vi "Check slice image.vi"(8 "Error in":errorcluster, 9 "Pause?":bool[](array[boolean]), 10 "image thickness":u32[](array[numeric]), 11 "slice thickness":u32[](array[numeric])) -> (0 "Error out":errorcluster, 5 "Exit?":bool)   [LabVIEW 2018]
uses:
  Controls/Queue Manager Actions.ctl
  Controls/MessagePacket.ctl
  Controls/FGV Actions.ctl
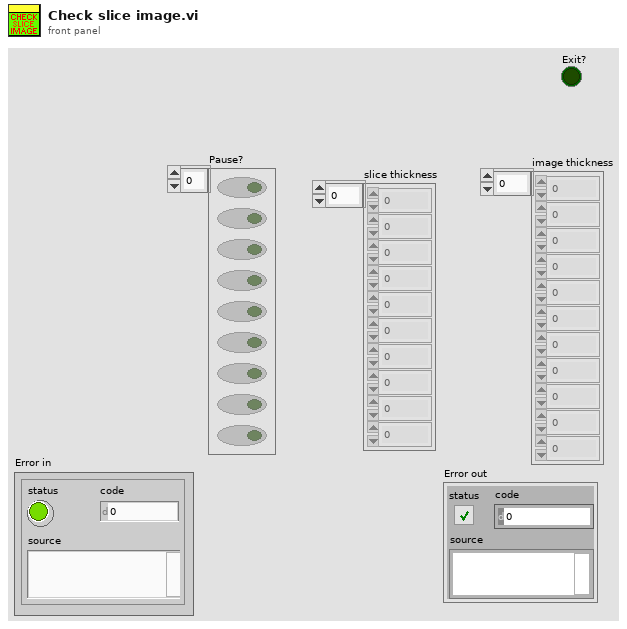
[diagram p1: front panel]
types:
  T1 = typedef "FGV Actions.ctl" = enum16{"Init", "Set", "Get", "Clear"}
  T2 = typedef "Queue Manager Actions.ctl" = enum16{"Init", "Enqueue", "Enqueue All", "Preview Queue", "Dequeue", "Get Status", "Flush Queue", "Flush All Queues", "Release All Queues", "Release Queue", "Enqueue at Opposite End"}
  T3 = typedef "MessagePacket.ctl" = cluster{"Message":string, "Parameter":variant}
  T4 = typedef "ScanType.ctl" = enum16{"Single Frame", "Continuous Frame", "ROI Line", "Vibratome", "Mosaic", "Mosaic + Slice"}
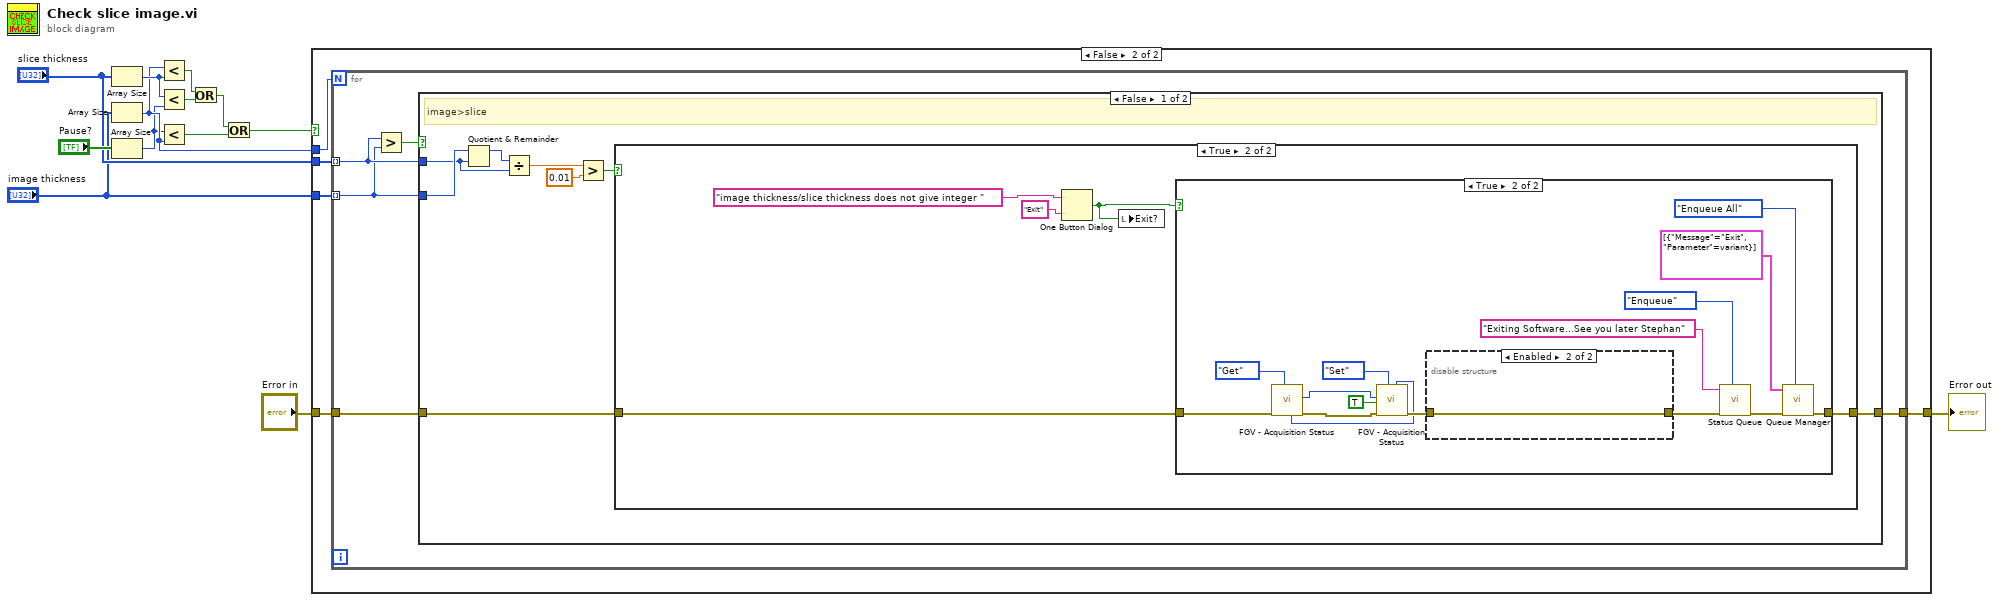
[diagram p0: block diagram]
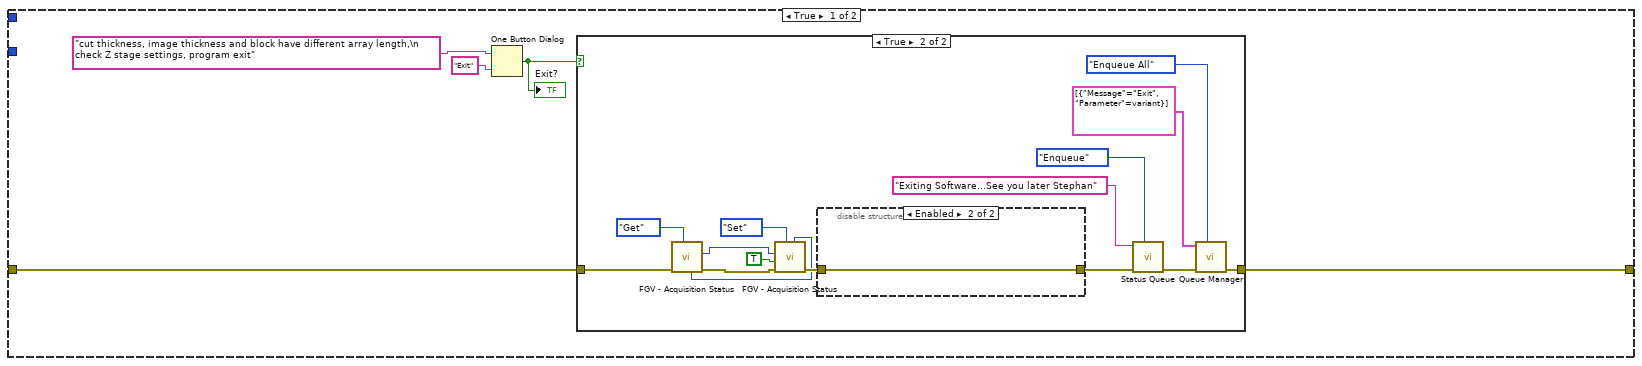
[diagram p2: hidden frame]
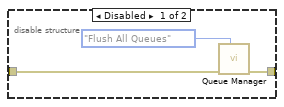
[diagram p4: hidden frame]
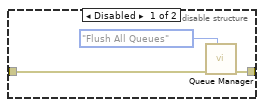
[diagram p7: hidden frame]
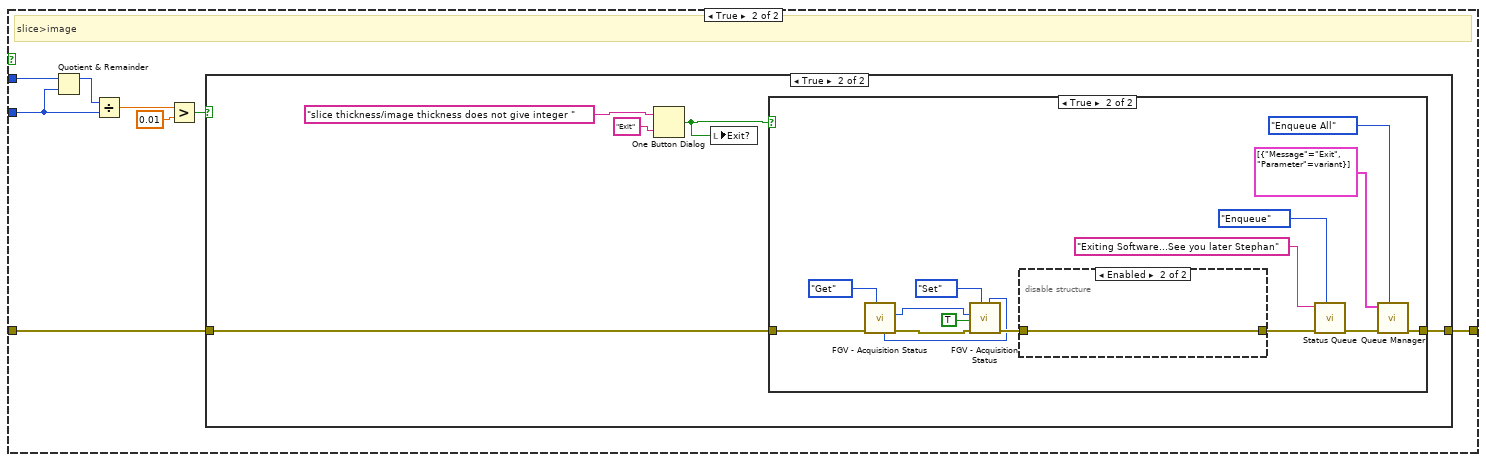
[diagram p8: hidden frame]
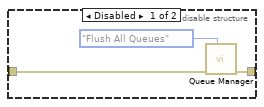
[diagram p11: hidden frame]
diagram:
  n1 = Array Size(array="slice thickness") -> (size(s)=w5:i32)
  n2 = Array Size(array="image thickness") -> (size(s)=w4:i32)
  n3 = Array Size(array="Pause?") -> (size(s)=w3:i32)
  n4 = Less?(x=w4, y=w5) -> (x < y?=w11:bool)
  n5 = Less?(x=w5, y=w3) -> (x < y?=w10:bool)
  n6 = Less?(x=w3, y=w4) -> (x < y?=w7:bool)
  n7 = Or(x=w11, y=w10) -> (x .or. y?=w8:bool)
  n8 = Or(x=w8, y=w7) -> (x .or. y?=w6:bool)
  n9 = case shown="False" w6 {
    tunnel: "Error in" -> [w15 w40]
    tunnel: [w14 w39] -> w12
    tunnel: w4 -> [_ w43]
    tunnel: "slice thickness" -> [_ w42]
    tunnel: "image thickness" -> [_ w41]
    frame True {
      n10 = One Button Dialog(message="cut thickness, image thickness and block have different array length,\n check Z stage settings, program exit", button name ("OK")="Exit") -> (true=w16:bool)
      "Exit?" <- w16
      n11 = case shown="True" w16 {
        tunnel: w15 -> [w19 w21]
        tunnel: [w19 w20] -> w14
        frame False {
        }
        frame True {
          n12 = call "FGV - Acquisition Status.vi"("Actions"=FGV_Actions."Get", "Error In"=w21) -> ("Error Out"=w26:errorcluster, "Scan Type [Out]"=w24:T4, "mem loc out"=w22:i32)  [unwired: 6 in, 1 out]
          n13 = call "FGV - Acquisition Status.vi"("mem loc"=w22, "Actions"=FGV_Actions."Set", "Error In"=w26, "Quit status"=TRUE, "Scan Type [In]"=w24) -> ("Error Out"=w25:errorcluster)  [unwired: 3 in, 3 out]
          n14 = disable-structure shown="Enabled" {
            disable-tunnel: [w36 w38] -> w29
            disable-tunnel: w25 -> [w35 w38]
            frame Disabled {
              n15 = call "Queue Manager.vi"("Action"=Queue_Manager_Actions."Flush All Queues", "Error In"=w35) -> ("Error Out"=w36:errorcluster)  [unwired: 5 in, 4 out]
            }
            frame Enabled {
            }
          }
          n16 = call "Status Queue.vi"("Action"=Queue_Manager_Actions."Enqueue", "Error In"=w29, "Status Message [In]"="Exiting Software...See you later Stephan") -> ("Error Out"=w31:errorcluster)  [unwired: 7 in, 1 out]
          n17 = call "Queue Manager.vi"("Action"=Queue_Manager_Actions."Enqueue All", "Error In"=w31, "Message Packet Array"=T3[] [{"Message"="Exit", "Parameter"=variant}] ("Message Packet [In]")) -> ("Error Out"=w20:errorcluster)  [unwired: 4 in, 4 out]
        }
      }
    }
    frame False {
      n18 = for {
        N: w43 -> [_]
        tunnel: w42 -> [w47] mode=indexing
        tunnel: w41 -> [w46] mode=indexing
        tunnel: w40 -> [w45]
        tunnel: [w44] -> w39
        n19 = Greater?(x=w47, y=w46) -> (0:w48:bool)
        n20 = case shown="False" w48 {
          tunnel: w47 -> [w50 w90]
          tunnel: w46 -> [w51 w85]
          tunnel: w45 -> [w52 w87]
          tunnel: [w49 w83] -> w44
          frame False {
            # "image>slice"
            n21 = Quotient & Remainder(x=w51, y=w50) -> (x-y*floor(x/y)=w54:u32)  [unwired: 1 out]
            n22 = Divide(x=w54, y=w50) -> (x/y=w53:dbl)
            n23 = Greater?(x=w53, y=0.01) -> (0:w55:bool)
            n24 = case shown="True" w55 {
              tunnel: w52 -> [w57 w60]
              tunnel: [w57 w59] -> w49
              frame False {
              }
              frame True {
                n25 = One Button Dialog(message="image thickness/slice thickness does not give integer ", button name ("OK")="Exit") -> (true=w58:bool)
                n26 = local write "Exit?"(w58) -> ()
                n27 = case shown="True" w58 {
                  tunnel: w60 -> [w63 w65]
                  tunnel: [w63 w64] -> w59
                  frame False {
                  }
                  frame True {
                    n28 = call "FGV - Acquisition Status.vi"("Actions"=FGV_Actions."Get", "Error In"=w65) -> ("Error Out"=w70:errorcluster, "Scan Type [Out]"=w68:T4, "mem loc out"=w66:i32)  [unwired: 6 in, 1 out]
                    n29 = call "FGV - Acquisition Status.vi"("mem loc"=w66, "Actions"=FGV_Actions."Set", "Error In"=w70, "Quit status"=TRUE, "Scan Type [In]"=w68) -> ("Error Out"=w69:errorcluster)  [unwired: 3 in, 3 out]
                    n30 = disable-structure shown="Enabled" {
                      disable-tunnel: [w80 w82] -> w73
                      disable-tunnel: w69 -> [w79 w82]
                      frame Disabled {
                        n31 = call "Queue Manager.vi"("Action"=Queue_Manager_Actions."Flush All Queues", "Error In"=w79) -> ("Error Out"=w80:errorcluster)  [unwired: 5 in, 4 out]
                      }
                      frame Enabled {
                      }
                    }
                    n32 = call "Status Queue.vi"("Action"=Queue_Manager_Actions."Enqueue", "Error In"=w73, "Status Message [In]"="Exiting Software...See you later Stephan") -> ("Error Out"=w75:errorcluster)  [unwired: 7 in, 1 out]
                    n33 = call "Queue Manager.vi"("Action"=Queue_Manager_Actions."Enqueue All", "Error In"=w75, "Message Packet Array"=T3[] [{"Message"="Exit", "Parameter"=variant}] ("Message Packet [In]")) -> ("Error Out"=w64:errorcluster)  [unwired: 4 in, 4 out]
                  }
                }
              }
            }
          }
          frame True {
            # "slice>image"
            n34 = Quotient & Remainder(x=w90, y=w85) -> (x-y*floor(x/y)=w86:u32)  [unwired: 1 out]
            n35 = Divide(x=w86, y=w85) -> (x/y=w84:dbl)
            n36 = Greater?(x=w84, y=0.01) -> (0:w88:bool)
            n37 = case shown="True" w88 {
              tunnel: w87 -> [w91 w93]
              tunnel: [w91 w92] -> w83
              frame False {
              }
              frame True {
                n38 = One Button Dialog(message="slice thickness/image thickness does not give integer ", button name ("OK")="Exit") -> (true=w94:bool)
                n39 = local write "Exit?"(w94) -> ()
                n40 = case shown="True" w94 {
                  tunnel: w93 -> [w97 w99]
                  tunnel: [w97 w98] -> w92
                  frame False {
                  }
                  frame True {
                    n41 = call "FGV - Acquisition Status.vi"("Actions"=FGV_Actions."Get", "Error In"=w99) -> ("Error Out"=w104:errorcluster, "Scan Type [Out]"=w102:T4, "mem loc out"=w100:i32)  [unwired: 6 in, 1 out]
                    n42 = call "FGV - Acquisition Status.vi"("mem loc"=w100, "Actions"=FGV_Actions."Set", "Error In"=w104, "Quit status"=TRUE, "Scan Type [In]"=w102) -> ("Error Out"=w103:errorcluster)  [unwired: 3 in, 3 out]
                    n43 = disable-structure shown="Enabled" {
                      disable-tunnel: [w114 w116] -> w107
                      disable-tunnel: w103 -> [w113 w116]
                      frame Disabled {
                        n44 = call "Queue Manager.vi"("Action"=Queue_Manager_Actions."Flush All Queues", "Error In"=w113) -> ("Error Out"=w114:errorcluster)  [unwired: 5 in, 4 out]
                      }
                      frame Enabled {
                      }
                    }
                    n45 = call "Status Queue.vi"("Action"=Queue_Manager_Actions."Enqueue", "Error In"=w107, "Status Message [In]"="Exiting Software...See you later Stephan") -> ("Error Out"=w109:errorcluster)  [unwired: 7 in, 1 out]
                    n46 = call "Queue Manager.vi"("Action"=Queue_Manager_Actions."Enqueue All", "Error In"=w109, "Message Packet Array"=T3[] [{"Message"="Exit", "Parameter"=variant}] ("Message Packet [In]")) -> ("Error Out"=w98:errorcluster)  [unwired: 4 in, 4 out]
                  }
                }
              }
            }
          }
        }
      }
    }
  }
  "Error out" <- w12
